vi "Measurement_input_panel.vi"(0 "OK":T4, 2 "setup":T5, 5 "Setup filename":string) -> (11 "Setup filename out":string, 12 "Analysis Info cluster":T7[](array[typedef])=[{"Colour"=0, "Inst type"=enum."Pitot-static tube", "Inst name"="Manometer voltage", "Symbol"="U", "Code name"="", "Extra Info"="U", "Inst Array"=enum."PWA", "U"=0.0, "u^2"=0.0, "u^3"=0.0, "u^4"=0.0, "Skew_u"=0.0, "Kurt_u"=0.0, "Sd Error in Mean"=0.0, "% u'/U"=0.0, "X"=0.0, "Y"=0.0, "Z"=0.0, "Timescale integral Estimate"=0.0, "Sd Error in Variance"=0.0, "Calib File"=path "", "Calib Constants"=[], "Output Position"=FALSE, "Stats"=enum."None", "Av Sampling Rate"=0.0, "Av No of Samples"=0.0, "Total Meas Time (s)"=0.0, "OrigChName"="", "Max value"=0.0, "Min value"=0.0, "Req Sample Rate Hz"=0.0, "Sync Delay Time (s)"=0.0, "Ch No"=0, "Device"="", "Use Latest Calib"=FALSE, "Port"="", "Metadata Ch Names"=[], "Metadata Ch Values"=[], "Label"="", "chState"=enum."Solo", "Point Drift"=0.0, "inputConfig"=""}, {"Colour"=0, "Inst type"=enum."Pitot-static tube", "Inst name"="Manometer voltage", "Symbol"="U", "Code name"="", "Extra Info"="U", "Inst Array"=enum."PWA", "U"=0.0, "u^2"=0.0, "u^3"=0.0, "u^4"=0.0, "Skew_u"=0.0, "Kurt_u"=0.0, "Sd Error in Mean"=0.0, "% u'/U"=0.0, "X"=0.0, "Y"=0.0, "Z"=0.0, "Timescale integral Estimate"=0.0, "Sd Error in Variance"=0.0, "Calib File"=path "", "Calib Constants"=[], "Output Position"=FALSE, "Stats"=enum."None", "Av Sampling Rate"=0.0, "Av No of Samples"=0.0, "Total Meas Time (s)"=0.0, "OrigChName"="", "Max value"=0.0, "Min value"=0.0, "Req Sample Rate Hz"=0.0, "Sync Delay Time (s)"=0.0, "Ch No"=0, "Device"="", "Use Latest Calib"=FALSE, "Port"="", "Metadata Ch Names"=[], "Metadata Ch Values"=[], "Label"="", "chState"=enum."Solo", "Point Drift"=0.0, "inputConfig"=""}, {"Colour"=0, "Inst type"=enum."Pitot-static tube", "Inst name"="Manometer voltage", "Symbol"="U", "Code name"="", "Extra Info"="U", "Inst Array"=enum."PWA", "U"=0.0, "u^2"=0.0, "u^3"=0.0, "u^4"=0.0, "Skew_u"=0.0, "Kurt_u"=0.0, "Sd Error in Mean"=0.0, "% u'/U"=0.0, "X"=0.0, "Y"=0.0, "Z"=0.0, "Timescale integral Estimate"=0.0, "Sd Error in Variance"=0.0, "Calib File"=path "", "Calib Constants"=[], "Output Position"=FALSE, "Stats"=enum."None", "Av Sampling Rate"=0.0, "Av No of Samples"=0.0, "Total Meas Time (s)"=0.0, "OrigChName"="", "Max value"=0.0, "Min value"=0.0, "Req Sample Rate Hz"=0.0, "Sync Delay Time (s)"=0.0, "Ch No"=0, "Device"="", "Use Latest Calib"=FALSE, "Port"="", "Metadata Ch Names"=[], "Metadata Ch Values"=[], "Label"="", "chState"=enum."Solo", "Point Drift"=0.0, "inputConfig"=""}] {"Kurt_u" format="%_3g"; "u^4" format="%_3g"; "u^3" format="%_3g"; "Sd Error in Variance" format="%_3g"; "u^2" format="%_3g"; "Sd Error in Mean" format="%_3g"; "U" format="%_3g"; "Sync Delay Time (s)" format="%.4f"; "Total Meas Time (s)" format="%_5g"; "Skew_u" format="%_3g"; "% u'/U" format="%_3g"})   [LabVIEW 2022 SP3]
uses:
  Controls/Inst_type.ctl
  Controls/portOrDev.ctl
  Controls/calType.ctl
  Controls/channelState.ctl
  Controls/DAQinputType.ctl
  Controls/Analysis_info_cluster.ctl
  Controls/Instrument_Array.ctl
  Controls/Setup.ctl
  Controls/ok_button.ctl
  Controls/Trigger_Mode.ctl
  Controls/PWA_Data.ctl
  File/Setup_Filetype.ctl
  Controls/Post_Process.ctl
  Controls/App_Global.ctl
  ADAM Client/Sub VIs/ADAM Controls/Channel_names.ctl
  ADAM Client/Sub VIs/Channel_State_Control.ctl
  <vilib>/Utility/error.llb/Trim Whitespace One-Sided.vi
  Globals/Meas_global.vi
  Globals/Trav_pos_global.vi
  Globals/LDA_global.vi
  Globals/Preference_global.vi
  Globals/Dynamic_call_global.ph.vi
panel:
  in  "DAQ Tigger Control?":bool
  in  "Port":refnum<visa-resource-name>="COM100"
  in  "Trigger mode":T1
  in  "Edit temp and Press":bool
  out "Abs Press":dbl=1013.0 caption="Absolute\nPressure" format="%.1fmBar"
  out "Temp":dbl=21.0 caption="Temperature" format="%.1fC"
  in  "Use  Analogue channel to software sync with LDA":bool
  in  "LDA_Setup":bool
  in  "Number of LDA Chs":i32 min=0 max=20
  in  "LDA data":enum16{"No LDA data", "Take LDA data"}(ring)=enum."Take LDA data"
  in  "PWA Data":T2
  out "Inst type":T3=enum."Propeller anemometer"
  in  "Select Plug Ins":bool
  out "XW Present?":bool
  out "Read Setup File?":bool
  out "Setup Paths":string[](array[string])
  in  "stop":bool
  out "Notes":string
  in  "Setup filename selector":u16(ring) items=["Current_Setup.xls", "GMU Source Q.xls", "7HP_Calibration.xls", "LDA_488_514_UV_Fast.xls", "LDA_488_514_UV_532_W Fast.xls", "LDA_488_514_UV_532_W.xls", "2HP_Boundary Layer.xls", "5H_Rake.xls"]
  in  "Cross wire":T6(ring)
  in  "No of Analogue inst":i32=1 caption="Number of Analogue Instruments"
  in  "Ch & spans choices":T13(array[cluster]) {"Fs" format="%#_pHz"; "syncDelay" format="%#_gms"; "Ch" min=0 step=1}
  # "Trigger Setup"
  # "Tunnel Conditions"
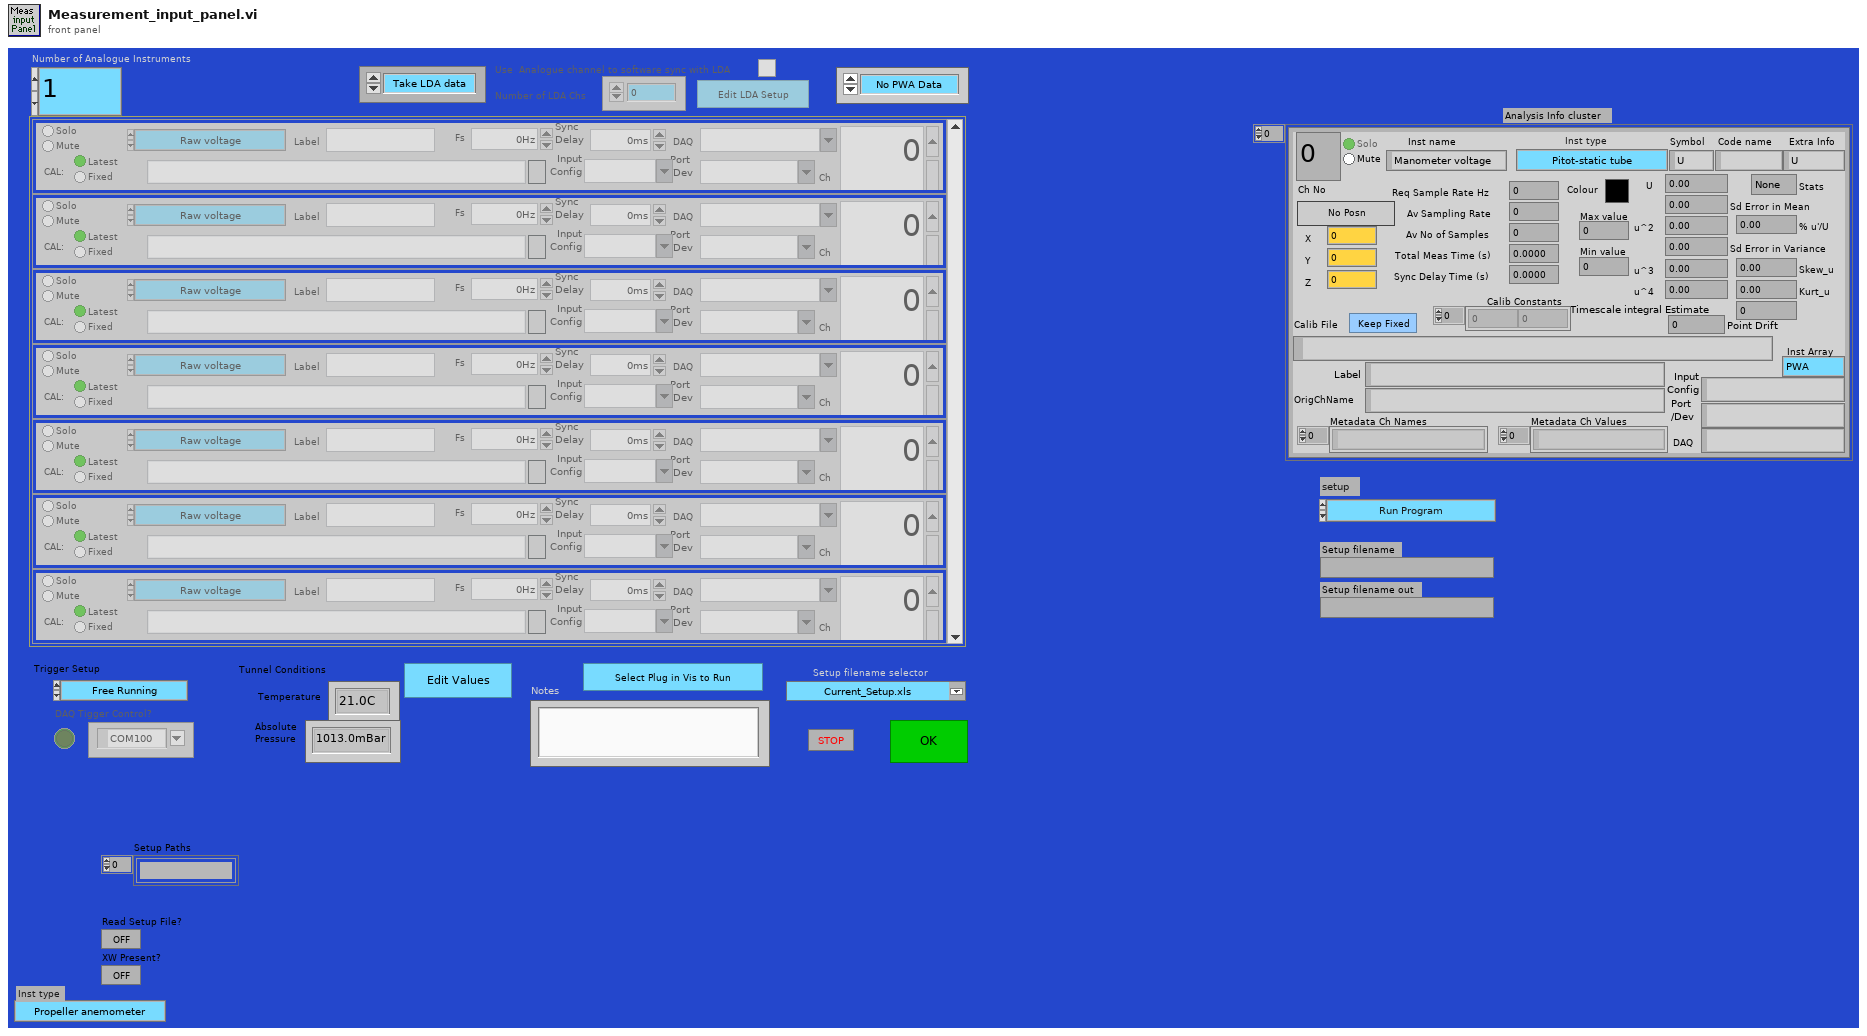
[diagram p1: front panel]
types:
  T1 = typedef "Trigger_Mode.ctl" = enum16{"Free Running", "Start on Trigger", "Trigger Every Block", "Trigger Every Sample"}
  T2 = typedef "PWA_Data.ctl" = enum16{"No PWA Data", "One Ch PWA"}
  T3 = typedef "Inst_type.ctl" = enum16{"Raw voltage", "Raw with zero offsetting", "Propeller anemometer", "Pressure Transducer", "Pitot-static tube", "Hot wire", "Cross wire 1", "Cross wire 2", "Generic Linear", "Generic Polynomial", "Generic BackPoly", "Fast FID", "Thermocouple", "Cold wire", "Pulsed Wire", "LDA Vel", "LDA Tran time", "LDA Arr time", "Microphone"}
  T4 = typedef "ok_button.ctl" = bool
  T5 = typedef "Setup.ctl" = enum16{"Run Program", "Show Setup", "Save Current Setup", "Setup Front Panel"}
  T6 = enum16{"2nd component as calculated", "2nd component multipled by -1"}
  T7 = typedef "Analysis_info_cluster.ctl" = cluster{"Colour":u32, "Inst type":T3, "Inst name":string, "Symbol":string, "Code name":string, "Extra Info":string, "Inst Array":T8, "U":dbl, "u^2":dbl, "u^3":dbl, "u^4":dbl, "Skew_u":dbl, "Kurt_u":dbl, "Sd Error in Mean":dbl, "% u'/U":dbl, "X":dbl, "Y":dbl, "Z":dbl, "Timescale integral Estimate":dbl, "Sd Error in Variance":dbl, "Calib File":path, "Calib Constants":dbl[], "Output Position":bool, "Stats":enum16{"None", "Basic", "Full"}, "Av Sampling Rate":dbl, "Av No of Samples":dbl, "Total Meas Time (s)":dbl, "OrigChName":string, "Max value":dbl, "Min value":dbl, "Req Sample Rate Hz":dbl, "Sync Delay Time (s)":dbl, "Ch No":i16, "Device":string, "Use Latest Calib":bool, "Port":string, "Metadata Ch Names":string[], "Metadata Ch Values":string[], "Label":string, "chState":T9, "Point Drift":dbl, "inputConfig":string}
  T8 = typedef "Instrument_Array.ctl" = enum16{"PWA", "LDA", "Analogue"}
  T9 = typedef "channelState.ctl" = enum32{"No Selection", "Solo", "Mute"}
  T10 = typedef "portOrDev.ctl" = string
  T11 = typedef "calType.ctl" = enum32{"Latest", "Fixed"}
  T12 = typedef "DAQinputType.ctl" = string
  T13 = cluster{"Type":T3, "Label":string, "DAQ":string, "Port":T10, "Ch":i32, "Cal":path, "calType":T11, "Fs":dbl, "syncDelay":dbl, "chState":T9, "inputConfig":T12}[]
  T14 = typedef "Post_Process.ctl" = enum16{"Take New Data", "Post Process Raw Data File"}
  T15 = typedef "Setup_Filetype.ctl" = enum16{"Measurement Setups", "Calibration Setups", "General", "Results File Plotter Setups", "Speed Calib Tweaks"}
  T16 = enum8{"Enabled", "Disabled", "Disabled and Grayed Out"}
  T17 = typedef "App_Global.ctl" = enum16{"Read Global", "Write to Global", "Initialise Array"}
  T18 = typedef "Channel_names.ctl" = enum16{"Active Only", "Active + Off", "All Channels", "Changeable Only", "Always Off", "Always On", "Always Off or On"}
  T19 = typedef "Channel_State_Control.ctl" = enum16{"Channel Name", "Channel Name Starts with", "Main Address"}
  T20 = enum16{"Zero or one", "One", "Zero or more", "One or more"}
  T21 = typedef "Meas input Cluster.ctl" = cluster{"Type":T3, "Label":string, "DAQ":string, "Port":T10, "Ch":i32, "Cal":path, "calType":T11, "Fs":dbl, "syncDelay":dbl, "chState":T9, "inputConfig":T12}
  T22 = typedef "LDA_Channel.ctl" = cluster{"Wavelength (nm)":dbl, "Vel Comp":string, "Max Velocity":dbl, "Min Velocity":dbl, "Max Record length":u16, "Signal gain (dB)":i16, "High voltage":i16, "Optics Conversion Factor":dbl, "Min Record length":u16, "Multiply Velocity by -1":bool, "Signal to Noise Ratio":string, "Validation Ratio":string, "Probe":string, "Laser":string, "BSA":string, "Lense":string, "Beam Separation (mm)":dbl, "Focal Length (mm)":dbl, "COLOUR":u32, "BSA IP":string, "Velocity Range (m/s)":dbl, "Centre Velocity (m/s)":dbl, "Unshifted mW":dbl, "Shifted mW":dbl, "Bandwidth Hz":dbl, "Req Sampling Rate Hz":dbl, "Ch":i32, "CenterFreq Hz":dbl, "Laser IP":string, "Sync Delay (s)":dbl}
  T23 = cluster{"Type":T3, "Label":string, "DAQ":string, "Port":T10, "Ch":i32, "Cal":path, "calType":T11, "Fs":dbl, "syncDelay":dbl, "chState":T9, "inputConfig":T12}
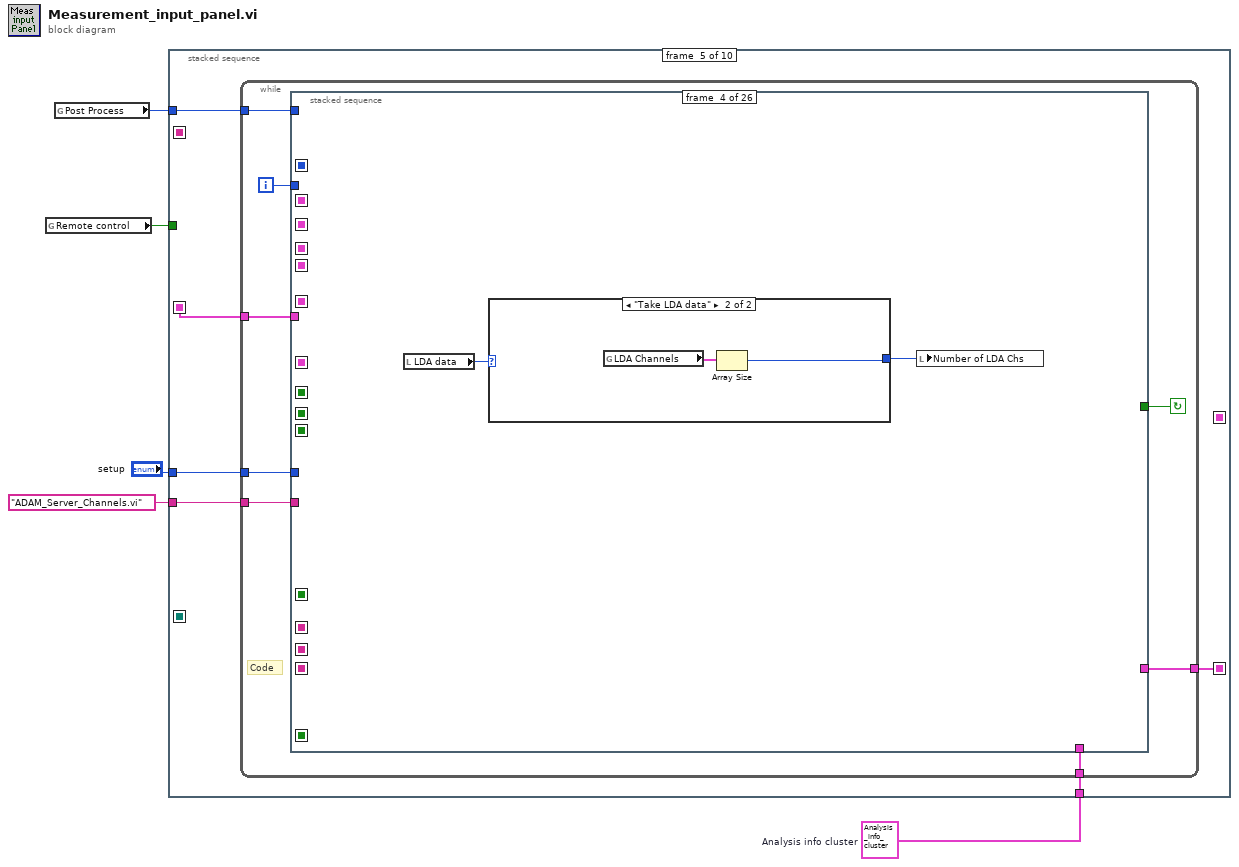
[diagram p0: block diagram]
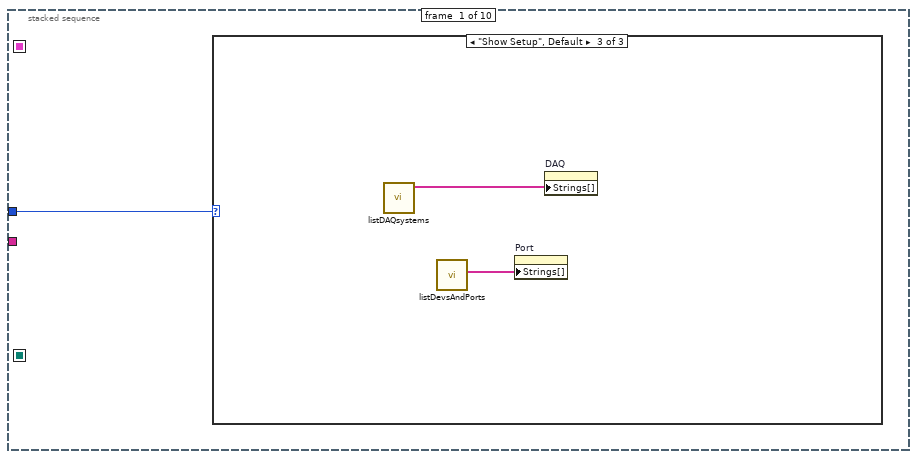
[diagram p2: hidden frame]
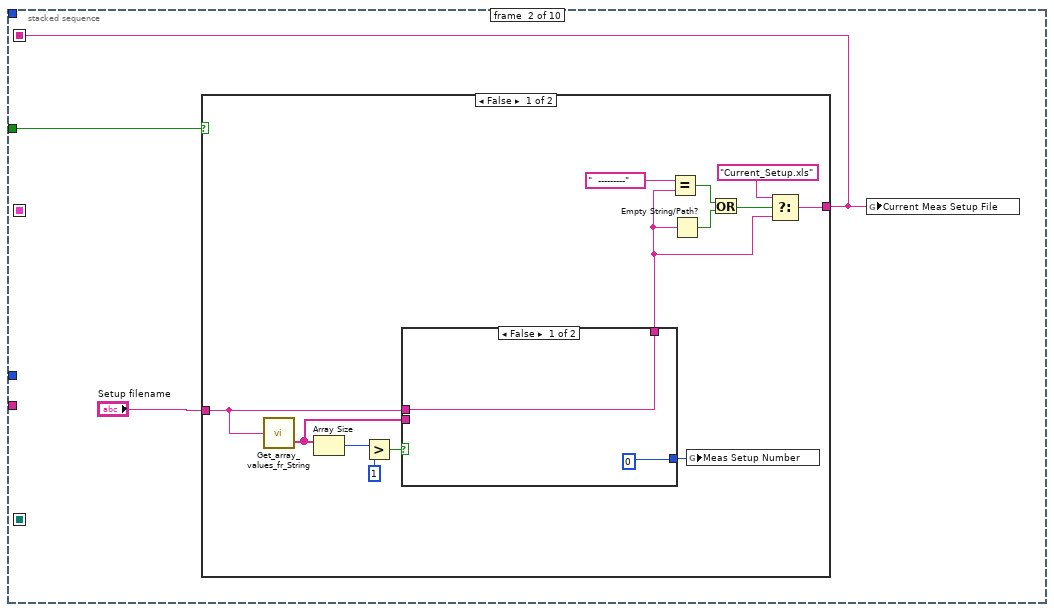
[diagram p5: hidden frame]
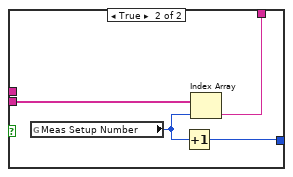
[diagram p6: hidden frame]
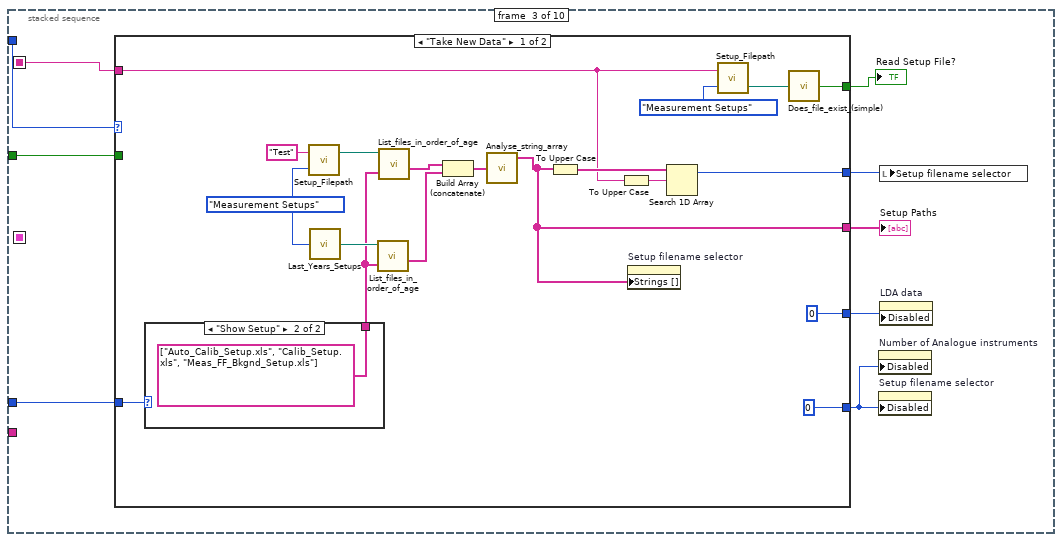
[diagram p8: hidden frame]
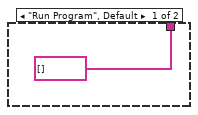
[diagram p9: hidden frame]
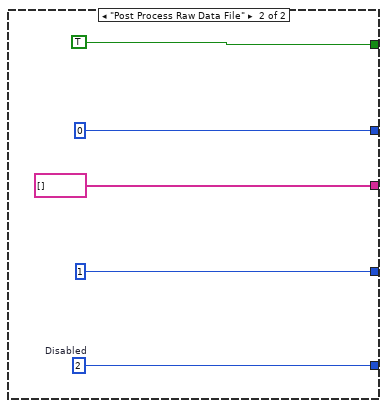
[diagram p10: hidden frame]
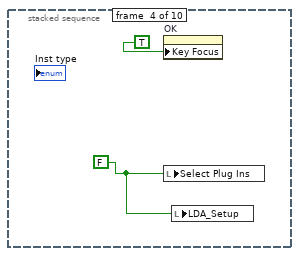
[diagram p11: hidden frame]
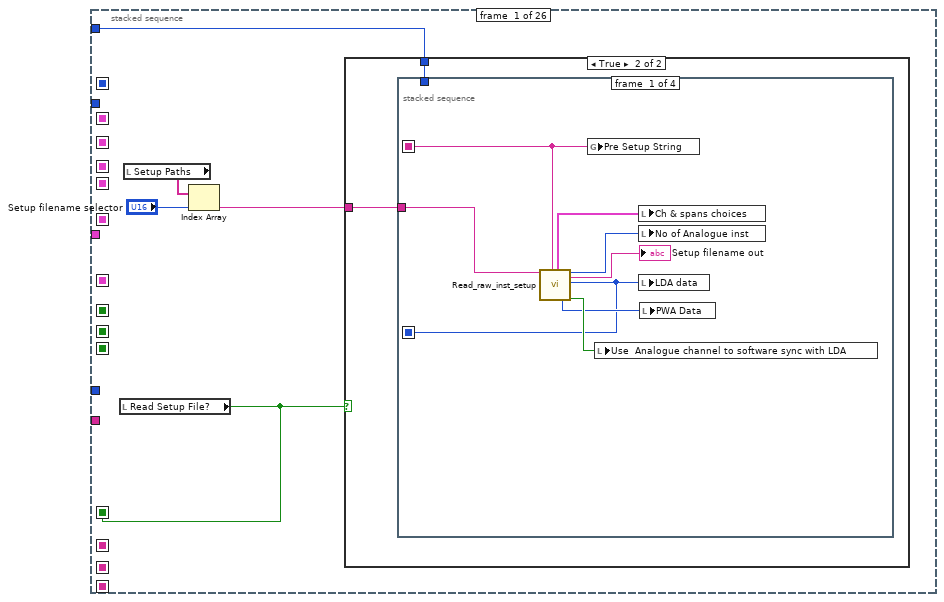
[diagram p12: hidden frame]
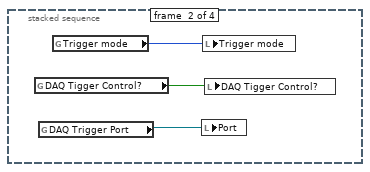
[diagram p14: hidden frame]
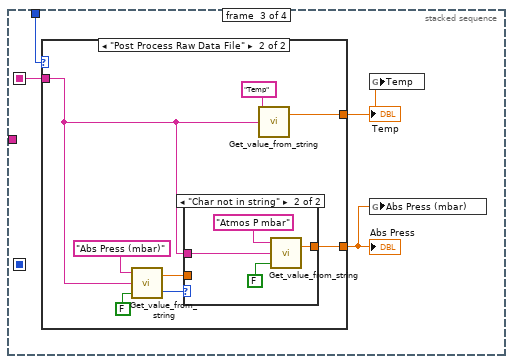
[diagram p15: hidden frame]
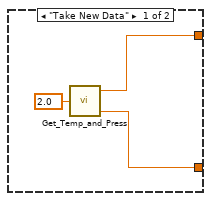
[diagram p16: hidden frame]
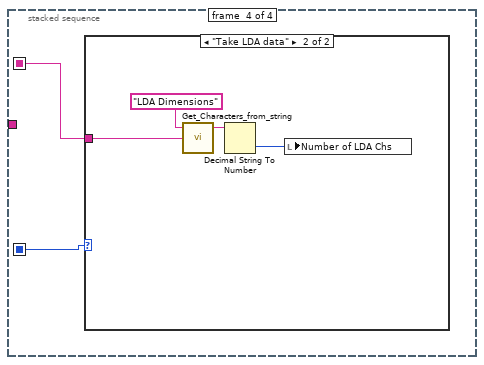
[diagram p18: hidden frame]
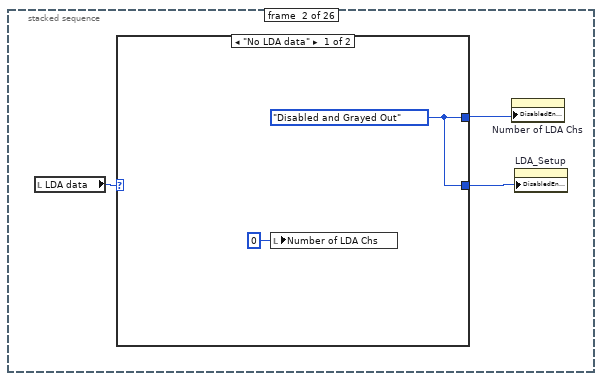
[diagram p20: hidden frame]
diagram:
  w1 = T7 {"Colour"=0, "Inst type"=enum."Pitot-static tube", "Inst name"="Manometer voltage", "Symbol"="U", "Code name"="", "Extra Info"="U", "Inst Array"=enum."PWA", "U"=0.0, "u^2"=0.0, "u^3"=0.0, "u^4"=0.0, "Skew_u"=0.0, "Kurt_u"=0.0, "Sd Error in Mean"=0.0, "% u'/U"=0.0, "X"=0.0, "Y"=0.0, "Z"=0.0, "Timescale integral Estimate"=0.0, "Sd Error in Variance"=0.0, "Calib File"=path "", "Calib Constants"=[], "Output Position"=FALSE, "Stats"=enum."None", "Av Sampling Rate"=0.0, "Av No of Samples"=0.0, "Total Meas Time (s)"=0.0, "OrigChName"="", "Max value"=0.0, "Min value"=0.0, "Req Sample Rate Hz"=0.0, "Sync Delay Time (s)"=0.0, "Ch No"=0, "Device"="", "Use Latest Calib"=FALSE, "Port"="", "Metadata Ch Names"=[], "Metadata Ch Values"=[], "Label"="", "chState"=enum."Solo", "Point Drift"=0.0, "inputConfig"=""}  # Analysis info cluster
  n1 = global read "Meas_global.vi" "Remote control"() -> (w3:bool)
  n2 = global read "Meas_global.vi" "Post Process"() -> (w5:T14)
  n3 = stacked-sequence {
    seq-local: [_ _ _ _ w74 _ _ _ _ _] -> [_ _ _ _ _ _ _ w765 _ _]
    seq-local: [_ w10 _ _ _ _ _ _ _ _] -> [_ _ w32 _ _ _ w630 _ _ _]
    seq-local: [_ _ _ _ w71 _ _ _ _ _] -> [_ _ _ _ _ _ _ _ _ w860]
    seq-local: [_ _ _ _ _ _ _ w764 _ _] -> [_ _ _ _ _ _ _ _ _ w861]
    seq-local: [_ _ _ _ _ _ _ _ w823 _] -> [_ _ _ _ _ _ _ _ _ w864]
    tunnel: w5 -> [_ _ w40 _ w73 _ _ w766 _ _]
    tunnel: "setup" -> [w6 _ w34 _ w72 _ w631 _ _ _]
    tunnel: w3 -> [_ w11 w33 _ _ _ _ _ _ _]
    tunnel: "ADAM_Server_Channels.vi" -> [_ _ _ _ w70 _ _ _ _ _]
    tunnel: w1 -> [_ _ _ _ w69 _ _ _ w826 _]
    frame #0 {
      n4 = case shown="\"Show Setup\", Default" w6 {
        frame "Run Program" {
        }
        frame "Setup Front Panel" {
        }
        frame "Show Setup", Default {
          n5 = call "listDAQsystems.vi"() -> ("DAQsystems"=w7:string[])  [unwired: 11 in]
          n6 = call "listDevsAndPorts.vi"() -> ("All Available Ports"=w8:string[])  [unwired: 11 in]
          n7 = property on="Port" class="CmbBox (strict)"("Strings[]"=w8) -> ()  [unwired: 2 in, 2 out]
          n8 = property on="DAQ" class="CmbBox"("Strings[]"=w7) -> ()  [unwired: 2 in, 2 out]
        }
      }
    }
    frame #1 {
      n9 = case shown="False" w11 {
        tunnel: [w23 w31] -> w10
        tunnel: "Setup filename" -> [w12 w31]
        frame False {
          n10 = call "Get_array_values_fr_String.vi"("String Value"=w12) -> ("String array"=w14:string[])  [unwired: 1 out]
          n11 = Array Size(array=w14) -> (size(s)=w18:i32)
          n12 = Greater?(x=w18, y=1) -> (0:w16:bool)
          n13 = case shown="False" w16 {
            tunnel: [w26 w29] -> w15
            tunnel: w12 -> [w26 _]
            tunnel: w14 -> [_ w30]
            tunnel: [0 w27] -> w13
            frame False {
            }
            frame True {
              n14 = global read "Trav_pos_global.vi" "Meas Setup Number"() -> (w28:i32)
              n15 = Increment(x=w28) -> (x+1=w27:i32)
              n16 = Index Array(array=w30, index=w28) -> (element=w29:string)
            }
          }
          n17 = Equal?(x="  ---------" ("f"), y=w15) -> (x = y?=w22:bool)
          n18 = Empty String/Path?(string/path=w15) -> (empty?=w21:bool)
          n19 = global write "Trav_pos_global.vi" "Meas Setup Number"(w13) -> ()
          n20 = Or(x=w22, y=w21) -> (x .or. y?=w19:bool)
          n21 = Select(t="Current_Setup.xls", s=w19, f=w15) -> (s? t:f=w23:string)
        }
        frame True {
        }
      }
      n22 = global write "Trav_pos_global.vi" "Current Meas Setup File"(w10) -> ()
    }
    frame #2 {
      n23 = case shown="\"Take New Data\"" w40 {
        tunnel: [w41 string[] []] -> w36
        tunnel: [w55 TRUE ("exists")] -> w35
        tunnel: [u8 0 ("Disabled") w63] -> w37
        tunnel: [u8 0 ("Disabled") u8 1 ("Disabled")] -> w39
        tunnel: w32 -> [w51 _]
        tunnel: [w58 0 ("index of element")] -> w38
        tunnel: w34 -> [w53 _]
        tunnel: w33 -> [_ _]
        frame "Take New Data" {
          w45 = Setup_Filetype."Measurement Setups" ("Setup File Type")
          n24 = case shown="\"Show Setup\"" w53 {
            tunnel: [string[] [] ("file names") string[] ["Auto_Calib_Setup.xls", "Calib_Setup.xls", "Meas_FF_Bkgnd_Setup.xls"] ("file names")] -> w43
            frame "Run Program", Default {
            }
            frame "Show Setup" {
            }
          }
          n25 = call "Setup_Filepath.vi"("Setup File Type"=w45, "Filename in"="Test") -> ("Directory"=w46:path)  [unwired: 1 out]
          n26 = call "Last_Years_Setups.vi"("Setup File Type"=w45) -> ("Directory"=w44:path)
          n27 = call "List_files_in_order_of_age.vi"("Files to Hide"=w43, "Folder"=w44) -> ("file names"=w48:string[])  [unwired: 9 in]
          n28 = call "List_files_in_order_of_age.vi"("Files to Hide"=w43, "Folder"=w46) -> ("file names"=w47:string[])  [unwired: 9 in]
          n29 = Build Array (concatenate)(w47, w48) -> (w42:string[])
          n30 = call "Analyse_string_array.vi"("String array"=w42) -> ("Unique strings"=w41:string[])  [unwired: 1 in, 1 out]
          n31 = To Upper Case(1:w41) -> (0:w57:string[])
          n32 = To Upper Case(1:w51) -> (0:w56:string)
          n33 = property on="Setup filename selector" class="Ring (strict)"("Strings []"=w41) -> ()  [unwired: 2 in, 2 out]
          n34 = Search 1D Array(1D array=w57, element=w56) -> (index of element=w58:i32)  [unwired: 1 out]
          n35 = call "Setup_Filepath.vi"("Setup File Type"=Setup_Filetype."Measurement Setups", "Filename in"=w51) -> ("Filename Out"=w50:path)  [unwired: 1 out]
          n36 = call "Does_file_exist_(simple).vi"("Pathname"=w50) -> ("exists?"=w55:bool)
        }
        frame "Post Process Raw Data File" {
          w63 = u8 2  # Disabled
        }
      }
      "Setup Paths" <- w36
      "Read Setup File?" <- w35
      n37 = property on="Number of Analogue instruments" class="DigNum (strict)"("Disabled"=w37) -> ()  [unwired: 2 in, 2 out]
      n38 = property on="Setup filename selector" class="Ring (strict)"("Disabled"=w37) -> ()  [unwired: 2 in, 2 out]
      n39 = local write "Setup filename selector"(w38) -> ()
      n40 = property on="LDA data" class="Enum (strict)"("Disabled"=w39) -> ()  [unwired: 2 in, 2 out]
    }
    frame #3 {
      w67 = FALSE ("Select Local ADAM Channels")
      n41 = property on="OK" class="Bool"("Key Focus"=TRUE) -> ()  [unwired: 2 in, 2 out]
      n42 = local write "Select Plug Ins"(w67) -> ()
      n43 = local write "LDA_Setup"(w67) -> ()
    }
    frame #4 {
      n44 = while {
        tunnel: w72 -> [w79]
        tunnel: w73 -> [w80]
        tunnel: [w82] -> w74
        tunnel: [w78] -> w71
        tunnel: w70 -> [w77]
        tunnel: w69 -> [w75]
        i -> [w76]
        stop <- w81 continue-if-true
        # "Code"
        n45 = stacked-sequence {
          seq-local: [_ _ _ _ _ _ _ _ _ _ _ w229 _ _ _ _ _ _ _ _ _ _ _ _ _ _] -> [_ _ _ _ _ _ _ _ _ _ _ _ _ _ w293 w346 _ _ _ _ _ _ _ _ _ _]
          seq-local: [_ _ _ _ "Ch & spans choices" _ _ _ _ _ _ _ _ _ _ _ _ _ _ _ _ _ _ _ _ _] -> [_ _ _ _ _ w168 _ _ w193 _ w225 w230 _ _ _ _ _ _ _ _ _ w566 _ _ _ _]
          seq-local: [_ _ _ _ _ _ _ _ w198 _ _ _ _ _ _ _ _ _ _ _ _ _ _ _ _ _] -> [_ _ _ _ _ _ _ _ _ _ _ w231 _ _ _ _ _ _ _ _ _ _ _ _ _ _]
          seq-local: [_ _ _ _ _ _ _ _ _ _ _ _ _ "OK" _ _ _ _ _ _ _ _ _ _ _ _] -> [_ _ _ _ _ _ _ _ _ _ _ _ _ _ w292 _ _ _ _ _ _ _ _ _ _ w595]
          seq-local: [_ _ _ _ _ _ _ _ _ _ _ _ _ _ _ _ w383 _ _ _ _ _ _ _ _ _] -> [_ _ _ _ _ _ _ _ _ _ _ _ _ _ _ _ _ _ w411 _ _ _ _ _ _ _]
          seq-local: [_ _ _ _ _ _ _ _ _ _ _ _ _ _ w297 _ _ _ _ _ _ _ _ _ _ _] -> [_ _ _ _ _ _ _ _ _ _ _ _ _ _ _ _ w385 _ _ _ _ _ _ _ _ _]
          seq-local: [_ _ _ _ _ _ _ _ _ _ _ _ _ _ _ w345 _ _ _ _ _ _ _ _ _ _] -> [_ _ _ _ _ _ _ _ _ _ _ _ _ _ _ _ w384 _ _ _ _ _ _ _ _ _]
          seq-local: [_ _ _ _ _ _ _ _ _ _ _ _ w287 _ _ _ _ _ _ _ _ _ _ _ _ _] -> [_ _ _ _ _ _ _ _ _ _ _ _ _ _ w294 _ _ _ _ _ _ _ _ _ _ w594]
          seq-local: [_ _ _ _ _ _ _ _ _ _ _ _ _ _ _ _ _ _ _ w458 _ _ _ _ _ _] -> [_ _ _ _ _ _ _ _ _ _ _ _ _ _ _ _ _ _ _ _ w536 _ _ _ _ _]
          seq-local: [_ _ _ _ _ _ _ _ _ _ _ _ _ _ _ _ _ _ _ w453 _ _ _ _ _ _] -> [_ _ _ _ _ _ _ _ _ _ _ _ _ _ _ _ _ _ _ _ w535 _ _ _ _ _]
          seq-local: [_ _ _ _ _ _ _ _ _ _ _ _ _ _ _ _ _ _ _ w457 _ _ _ _ _ _] -> [_ _ _ _ _ _ _ _ _ _ _ _ _ _ _ _ _ _ _ _ w534 _ _ _ _ _]
          seq-local: [w83 _ _ _ _ _ _ _ _ _ _ _ _ _ _ _ _ _ _ _ _ _ _ _ _ _] -> [_ _ _ _ _ _ _ _ _ _ _ _ _ _ _ _ _ _ _ _ w532 _ _ _ _ _]
          seq-local: [_ _ _ _ _ _ _ _ _ _ _ _ _ _ _ _ _ _ w412 _ _ _ _ _ _ _] -> [_ _ _ _ _ _ _ _ _ _ _ _ _ _ _ _ _ _ _ w455 _ w567 _ w570 _ w587]
          seq-local: [_ _ _ _ _ _ _ _ _ _ _ _ _ _ _ _ _ w403 _ _ _ _ _ _ _ _] -> [_ _ _ _ _ _ _ _ _ _ _ _ _ _ _ _ _ _ w413 _ _ _ _ _ _ _]
          seq-local: [_ _ _ _ _ _ _ _ _ _ _ _ _ _ _ _ _ _ _ w454 _ _ _ _ _ _] -> [_ _ _ _ _ _ _ _ _ _ _ _ _ _ _ _ _ _ _ _ w530 _ _ _ _ _]
          tunnel: [_ _ _ _ _ _ _ _ _ _ _ _ _ _ _ _ w383 _ _ _ _ _ _ _ _ _] -> w82
          tunnel: [_ _ _ _ _ _ _ _ _ _ _ _ _ _ w295 _ _ _ _ _ _ _ _ _ _ _] -> w81
          tunnel: w80 -> [w85 _ _ _ _ _ w174 _ _ _ _ _ w288 _ _ w344 _ w409 _ _ _ _ _ _ _ _]
          tunnel: w79 -> [_ _ _ _ _ w167 _ w181 _ _ _ _ _ _ _ _ w386 _ _ _ _ _ _ _ _ _]
          tunnel: [_ _ _ _ _ _ _ _ _ _ _ _ _ _ _ _ _ _ _ _ w533 _ _ _ _ _] -> w78
          tunnel: w77 -> [_ _ _ _ _ _ _ _ _ _ _ _ _ _ w291 _ _ w406 w414 _ _ _ _ _ _ _]
          tunnel: w76 -> [_ _ _ _ _ _ _ _ _ _ _ _ _ _ _ _ _ _ _ _ _ _ _ _ _ _]
          tunnel: w75 -> [_ _ _ _ _ _ _ _ _ _ _ _ _ _ _ _ _ _ _ _ w531 _ _ _ _ _]
          frame #0 {
            n46 = local read "Read Setup File?"() -> (w83:bool)
            n47 = local read "Setup Paths"() -> (w87:string[])
            n48 = Index Array(array=w87, index="Setup filename selector") -> (element=w84:string)
            n49 = case shown="True" w83 {
              tunnel: w84 -> [_ w89]
              tunnel: w85 -> [_ w88]
              frame False {
              }
              frame True {
                n50 = stacked-sequence {
                  seq-local: [w94 _ _ _] -> [_ _ w103 w121]
                  seq-local: [w92 _ _ _] -> [_ _ _ w122]
                  tunnel: w89 -> [w95 _ _ _]
                  tunnel: w88 -> [_ _ w104 _]
                  frame #0 {
                    n51 = call "Read_raw_inst_setup.vi"("Setup file"=w95) -> ("Setup string"=w94:string, "Ch & spans choices"=w91:T21[], "PWA Data"=w93:T2, "Number of Analogue instruments"=w97:i32, "Setup filename out"=→"Setup filename out":string, "LDA data"=w92:enum16{"No LDA data", "Take LDA data"}, "Use Analogue channel to software sync with LDA"=w96:bool)  [unwired: 12 out]
                    n52 = global write "Meas_global.vi" "Pre Setup String"(w94) -> ()
                    n53 = local write "Use  Analogue channel to software sync with LDA"(w96) -> ()
                    n54 = local write "Ch & spans choices"(w91) -> ()
                    n55 = local write "No of Analogue inst"(w97) -> ()
                    n56 = local write "LDA data"(w92) -> ()
                    n57 = local write "PWA Data"(w93) -> ()
                  }
                  frame #1 {
                    n58 = global read "Meas_global.vi" "DAQ Tigger Control?"() -> (w98:bool)
                    n59 = global read "Meas_global.vi" "DAQ Trigger Port"() -> (w99:refnum<visa-resource-name>)
                    n60 = global read "Meas_global.vi" "Trigger mode"() -> (w100:T1)
                    n61 = local write "Port"(w99) -> ()
                    n62 = local write "Trigger mode"(w100) -> ()
                    n63 = local write "DAQ Tigger Control?"(w98) -> ()
                  }
                  frame #2 {
                    n64 = case shown="\"Post Process Raw Data File\"" w104 {
                      tunnel: w103 -> [_ w110]
                      tunnel: [w105 w109] -> w101
                      tunnel: [w106 w108] -> w102
                      frame "Take New Data" {
                        n65 = call "Get_Temp_and_Press.vi"("Averaging time (mins)"=2.0) -> ("Abs Press (mbar)"=w105:dbl, "Temperature"=w106:dbl)  [unwired: 3 out]
                      }
                      frame "Post Process Raw Data File" {
                        n66 = call "Get_value_from_string.vi"("Show Dialog?"=FALSE, "Input string"=w110, "Variable name"="Abs Press (mbar)") -> ("Status"=w114:enum16{"Char in string", "Char not in string"}, "Value"=w113:dbl)
                        n67 = case shown="\"Char not in string\"" w114 {
                          tunnel: [w116 w119] -> w109
                          tunnel: w113 -> [w116 _]
                          tunnel: w110 -> [_ w118]
                          frame "Char in string" {
                          }
                          frame "Char not in string" {
                            n68 = call "Get_value_from_string.vi"("Show Dialog?"=FALSE, "Input string"=w118, "Variable name"="Atmos P mbar") -> ("Value"=w119:dbl)  [unwired: 1 out]
                          }
                        }
                        n69 = call "Get_value_from_string.vi"("Input string"=w110, "Variable name"="Temp") -> ("Value"=w108:dbl)  [unwired: 1 in, 1 out]
                      }
                    }
                    "Abs Press" <- w101
                    "Temp" <- w102
                    n70 = global write "Meas_global.vi" "Temp"(w102) -> ()
                    n71 = global write "Meas_global.vi" "Abs Press (mbar)"(w101) -> ()
                  }
                  frame #3 {
                    n72 = case shown="\"Take LDA data\"" w122 {
                      tunnel: w121 -> [_ w124]
                      frame "No LDA data" {
                      }
                      frame "Take LDA data" {
                        n73 = call "Get_Characters_from_string.vi"("Input string"=w124, "Variable name"="LDA Dimensions") -> ("Value"=w126:string)  [unwired: 1 in, 1 out]
                        n74 = Decimal String To Number(string=w126) -> (number=w123:i32)  [unwired: 2 in, 1 out]
                        n75 = local write "Number of LDA Chs"(w123) -> ()
                      }
                    }
                  }
                }
              }
            }
          }
          frame #1 {
            n76 = local read "LDA data"() -> (w129:enum16{"No LDA data", "Take LDA data"})
            n77 = case shown="\"No LDA data\"" w129 {
              tunnel: [w130 w132] -> w128
              tunnel: [w130 w132] -> w127
              frame "No LDA data" {
                w130 = T16."Disabled and Grayed Out" ("Disabled")
                n78 = local write "Number of LDA Chs"(i16 0 ("Number of LDA Chs")) -> ()
              }
              frame "Take LDA data" {
                w132 = T16."Enabled" ("Disabled")
              }
            }
            n79 = property on="Number of LDA Chs" class="DigNum (strict)"("DisabledEnum"=w128) -> ()  [unwired: 2 in, 2 out]
            n80 = property on="LDA_Setup" class="Bool (strict)"("DisabledEnum"=w127) -> ()  [unwired: 2 in, 2 out]
          }
          frame #2 {
            n81 = case shown="True" "LDA_Setup" {
              frame False {
              }
              frame True {
                n82 = global read "Meas_global.vi" "Pre Setup String"() -> (w137:string)
                n83 = call "Get_value_from_string.vi"("Input string"=w137, "Variable name"="BSA 1 Calibration factor") -> ("Status"=w136:enum16{"Char in string", "Char not in string"})  [unwired: 1 in, 1 out]
                n84 = local write "LDA_Setup"(FALSE ("LDA_Setup")) -> ()
                n85 = Equal?(x=w136, y=enum16{"Char in string", "Char not in string"}."Char in string" ("Status")) -> (x = y?=w134:bool)
                n86 = call "Edit LDA Setup.vi"("LDA info in Setup File?"=w134) -> ()  [unwired: 11 in]
              }
            }
          }
          frame #3 {
            n87 = local read "LDA data"() -> (w141:enum16{"No LDA data", "Take LDA data"})
            n88 = case shown="\"Take LDA data\"" w141 {
              tunnel: [0 ("Number of LDA Chs") w143] -> w140
              frame "No LDA data" {
              }
              frame "Take LDA data" {
                n89 = global read "LDA_global.vi" "LDA Channels"() -> (w144:T22[])
                n90 = Array Size(array=w144) -> (size(s)=w143:i32)
              }
            }
            n91 = local write "Number of LDA Chs"(w140) -> ()
          }
          frame #4 {
            n92 = local read "Read Setup File?"() -> (w150:bool)
            n93 = local read "Trigger mode"() -> (w148:T1)
            n94 = case shown="True" w150 {
              frame False {
              }
              frame True {
                n95 = global read "Meas_global.vi" "Pre Setup String"() -> (w159:string)
                n96 = call "Get_Characters_from_string.vi"("Input string"=w159, "Variable name"="Invert Second Component") -> ("Status"=w158:enum16{"Char in string", "Char not in string"}, "Value"=w157:string)  [unwired: 1 in]
                n97 = case shown="\"Char in string\"" w158 {
                  tunnel: w157 -> [w166 _]
                  frame "Char in string" {
                    n98 = Equal?(x="TRUE", y=w166) -> (x = y?=w162:bool)
                    n99 = Select(t=T6."2nd component multipled by -1" ("Cross wire/LDA"), s=w162, f=T6."2nd component as calculated" ("Cross wire/LDA")) -> (s? t:f=w164:T6)
                    n100 = local write "Cross wire"(w164) -> ()
                  }
                  frame "Char not in string" {
                  }
                }
              }
            }
            n101 = case shown="Default" w148 {
              tunnel: [w151 w152] -> w147
              tunnel: [w151 w153] -> w146
              tunnel: "DAQ Tigger Control?" -> [_ w154]
              frame "Free Running" {
                w151 = T16."Disabled and Grayed Out" ("Disabled")
              }
              frame Default {
                w152 = T16."Enabled" ("Disabled")
                n102 = case shown="False" w154 {
                  tunnel: [T16."Disabled and Grayed Out" ("Disabled") w156] -> w153
                  tunnel: w152 -> [_ w156]
                  frame False {
                  }
                  frame True {
                  }
                }
              }
            }
            n103 = property on="Port" class="VISAName"("DisabledEnum"=w146) -> ()  [unwired: 2 in, 2 out]
            n104 = property on="DAQ Tigger Control?" class="Bool (strict)"("DisabledEnum"=w147) -> ()  [unwired: 2 in, 2 out]
          }
          frame #5 {
            n105 = case shown="\"Show Setup\"" w167 {
              tunnel: w168 -> [_ w171]
              frame "Run Program", Default {
              }
              frame "Show Setup" {
                n106 = for {
                  tunnel: w171 -> [w173] mode=indexing
                  tunnel: [w172] -> w170 mode=indexing
                  n107 = Unbundle By Name(w173) -> ("DAQ"=w172:string)
                }
                n108 = call "Analyse_string_array.vi"("String array"=w170) -> ("Unique strings"=w169:string[])  [unwired: 1 in, 1 out]
                n109 = global write "Meas_global.vi" "Acquisition_Plug_Ins to Run"(w169) -> ()
              }
            }
          }
          frame #6 {
            n110 = case shown="True" "Edit temp and Press" {
              tunnel: w174 -> [_ w176]
              frame False {
              }
              frame True {
                n111 = case shown="\"Take New Data\"" w176 {
                  frame "Take New Data" {
                    n112 = stacked-sequence {
                      frame #0 {
                        w177 = TRUE  # Wait until done
                        n113 = call "Run_Enter_Temp.vi"("Wait until done"=w177) -> ()  [unwired: 1 out]
                      }
                      frame #1 {
                        n114 = call "Get_Temp_and_Press.vi"("Averaging time (mins)"=2.0) -> ("Abs Press (mbar)"=w178:dbl, "Temperature"=w179:dbl)  [unwired: 3 out]
                        n115 = local write "Abs Press"(w178) -> ()
                        n116 = local write "Temp"(w179) -> ()
                      }
                    }
                  }
                  frame "Post Process Raw Data File" {
                  }
                }
              }
            }
          }
          frame #7 {
            n117 = case shown="True" "Select Plug Ins" {
              tunnel: w181 -> [_ w183]
              frame False {
              }
              frame True {
                n118 = stacked-sequence {
                  tunnel: w183 -> [w184 _]
                  frame #0 {
                    w188 = TRUE  # Show Panel?
                    n119 = global read "Meas_global.vi" "Pre Setup String"() -> (w187:string)
                    n120 = local write "Select Plug Ins"(FALSE ("Select Local ADAM Channels")) -> ()
                    n121 = call "Choose_Plug_In_to_Run.vi"("setup"=w184, "Show Panel?"=w188, "Setup String In"=w187) -> ("Setup String Out"=w186:string)  [unwired: 1 out]
                    n122 = global write "Meas_global.vi" "Pre Setup String"(w186) -> ()
                  }
                  frame #1 {
                    n123 = Current VI's Path() -> (path=w190:path)
                    n124 = call "Open_Close_Front_Panel.ph.vi"("openWindow (T)"=TRUE ("Front Panel Window:Open"), "VI path"=w190) -> ()  [unwired: 1 in, 1 out]
                  }
                }
              }
            }
          }
          frame #8 {
            n125 = Initialize Array(0) -> (w200:i32[])  [unwired: 1 out]
            n126 = for {
              shift-right: [w205] -> w196
              shift-left: w200 -> [w206]
              tunnel: [w204] -> w194 mode=indexing
              tunnel: w193 -> [w203] mode=indexing
              n127 = Unbundle By Name(w203) -> ("Type"=w202:T3)
              n128 = case shown="\"LDA Vel\"" w202 {
                tunnel: w206 -> [w210 w214 w216 w220]
                tunnel: [w209 w213 w216 w219] -> w205
                tunnel: [FALSE TRUE FALSE FALSE] -> w204
                frame "Propeller anemometer", Default {
                  n129 = Build Array (concatenate)(w210, 1) -> (w209:i32[])
                }
                frame "Cross wire 1" {
                  n130 = Build Array (concatenate)(w214, 2) -> (w213:i32[])
                }
                frame "Cross wire 2" {
                }
                frame "LDA Vel" {
                  n131 = Build Array (concatenate)(w220, 1) -> (w219:i32[])
                }
              }
            }
            n132 = Or Array Elements(Boolean array=w194) -> (logical OR=→"XW Present?":bool)
            n133 = Build Array (concatenate)(w196, 1) -> (w195:i32[])
            n134 = Array Subset(array=w195, length="No of Analogue inst") -> (w199:i32[])  [unwired: 1 in]
            n135 = Add Array Elements(numeric array=w199) -> (sum=w198:i32)
          }
          frame #9 {
            "Notes" <- ""
          }
          frame #10 {
            n136 = Array Size(array=w225) -> (size(s)=w224:i32)
            n137 = Not Equal To 0?(x=w224) -> (x != 0?=w223:bool)
            n138 = case shown="True" w223 {
              tunnel: [enum16{"No Analogue data", "Take Analogue data"}."No Analogue data" ("Analogue data") enum16{"No Analogue data", "Take Analogue data"}."Take Analogue data" ("Analogue data")] -> w222
              frame False {
              }
              frame True {
              }
            }
            n139 = global write "Meas_global.vi" "Analogue data"(w222) -> ()
          }
          frame #11 {
            n140 = Index Array(array=w230, index=0) -> (element=w235:T23)
            n141 = Initialize Array(w235) -> (w233:T13)  [unwired: 1 out]
            n142 = Build Array (concatenate)(w230, w235) -> (w234:T13)
            n143 = for {
              N: w231 -> [_]
              tunnel: w234 -> [w243] mode=indexing
              shift-right: [w244] -> w229
              shift-left: w233 -> [w238]
              tunnel: Inst_type."Cross wire 2" ("Inst type") -> [w236]
              shift-right: [w242] -> _
              shift-left: _ -> [w241]
              tunnel: w234 -> [w240]
              n144 = Unbundle By Name(w243) -> ("Type"=w242:T3)
              n145 = Array Size(array=w238) -> (size(s)=w237:i32)
              n146 = Increment(x=w237) -> (x+1=w239:i32)
              n147 = case shown="\"Cross wire 1\"" w242 {
                tunnel: [w252 w272 w284] -> w244
                tunnel: w238 -> [w253 w274 w286]
                tunnel: w243 -> [w249 w275 w285]
                tunnel: w236 -> [w251 w279 _]
                tunnel: w241 -> [_ w278 _]
                tunnel: w240 -> [w256 _ _]
                tunnel: w239 -> [w255 _ _]
                frame "Cross wire 1" {
                  n148 = Index Array(array=w256, index=w255) -> (element=w250:T23)
                  n149 = Unbundle By Name(w250) -> ("Type"=w254:T3, "syncDelay"=w247:dbl, "Ch"=w246:i32, "Label"=w245:string)
                  n150 = Unbundle By Name(w249) -> ("Cal"=w248:path)
                  n151 = case shown="\"Generic Linear\", Default" w254 {
                    tunnel: w253 -> [w265 w271]
                    tunnel: [w264 w270] -> w252
                    tunnel: w251 -> [w258 w266]
                    tunnel: w248 -> [w263 w269]
                    tunnel: w249 -> [w261 w267]
                    tunnel: w247 -> [w260 _]
                    tunnel: w246 -> [w259 _]
                    tunnel: w245 -> [w257 _]
                    frame "Cross wire 2" {
                      n152 = Bundle By Name(cluster=w261, "Cal"=w263, "Type"=w258, "syncDelay"=w260, "Ch"=w259, "Label"=w257) -> (w262:T23)
                      n153 = Build Array (concatenate)(w265, w261, w262) -> (w264:T13)
                    }
                    frame "Generic Linear", Default {
                      n154 = Bundle By Name(cluster=w267, "Cal"=w269, "Type"=w266) -> (w268:T23)
                      n155 = Build Array (concatenate)(w271, w267, w268) -> (w270:T13)
                    }
                  }
                }
                frame "Cross wire 2" {
                  n156 = Decrement(x=w279) -> (x-1=w277:T3)
                  n157 = Equal?(x=w277, y=w278) -> (x = y?=w276:bool)
                  n158 = Bundle By Name(cluster=w275, "Type"=w277) -> (w273:T23)
                  n159 = case shown="False" w276 {
                    tunnel: w274 -> [w282 w283]
                    tunnel: w273 -> [w281 _]
                    tunnel: [w280 w283] -> w272
                    frame False {
                      n160 = Build Array (concatenate)(w282, w281) -> (w280:T13)
                    }
                    frame True {
                    }
                  }
                }
                frame "Generic Linear", Default {
                  n161 = Build Array (concatenate)(w286, w285) -> (w284:T13)
                }
              }
            }
          }
          frame #12 {
            n162 = Equal?(x=w288, y=Post_Process."Take New Data" ("Post Process")) -> (x = y?=w287:bool)
          }
          frame #13 {
          }
          frame #14 {
            n163 = And(x=w294, y=w292) -> (x .and. y?=w296:T4)
            n164 = case shown="True" w296 {
              tunnel: w293 -> [_ w306]
              tunnel: [FALSE w305] -> w297
              tunnel: [w298 w304] -> w295
              tunnel: w292 -> [w299 _]
              tunnel: w291 -> [_ w301]
              frame False {
                n165 = Not(x=w299) -> (.not. x?=w298:T4)
              }
              frame True {
                n166 = for {
                  shift-right: [w331] -> _
                  shift-left: string[] [] -> [w330]
                  tunnel: w306 -> [w329] mode=indexing
                  tunnel: [w321] -> w307 mode=indexing
                  shift-right: [w328] -> _
                  shift-left: path[] [] -> [w327]
                  tunnel: w301 -> [w309]
                  n167 = Unbundle By Name(w329) -> ("Type"=w326:T3, "Cal"=w317:path, "DAQ"=w310:string)
                  n168 = call "Full Channel ID.vi"("Cluster"=w329) -> ("String"=w314:string)
                  n169 = Equal?(x=w310, y=w309) -> (x = y?=w308:bool)
                  n170 = Search 1D Array(1D array=w330, element=w314) -> (index of element=w315:i32)  [unwired: 1 out]
                  n171 = Equal?(x=Inst_type."Fast FID" ("Inst type"), y=w326) -> (x = y?=w320:bool)
                  n172 = Less Than 0?(x=w315) -> (x < 0?=w313:bool)
                  n173 = Empty String/Path?(string/path=w314) -> (empty?=w312:bool)
                  n174 = Search 1D Array(1D array=w327, element=w317) -> (index of element=w324:i32)  [unwired: 1 out]
                  n175 = Compound Arithmetic op=OR(w312, w313, w308) -> (w311:bool)
                  n176 = Empty String/Path?(string/path=w317) -> (empty?=w316:bool)
                  n177 = Greater Or Equal To 0?(x=w324) -> (x >= 0?=w319:bool)
                  n178 = case shown="False" w311 {
                    tunnel: w314 -> [w342 _]
                    tunnel: [w338 FALSE ("true")] -> w323
                    frame False {
                      n179 = Format Into String(format string="The Channel %s appears more than once", w342) -> (resulting string=w340:string)  [unwired: 2 in, 1 out]
                      n180 = One Button Dialog(message=w340, button name ("OK")="Ok") -> (true=w338:bool)
                    }
                    frame True {
                    }
                  }
                  n181 = Compound Arithmetic op=AND(w319, w320, invert w316) -> (w318:bool)
                  n182 = case shown="True" w318 {
                    tunnel: [w333 FALSE ("true")] -> w322
                    tunnel: w317 -> [w332 _]
                    frame True {
                      n183 = Format Into String(format string="Calibration file %s is used more than once.", w332) -> (resulting string=w335:string)  [unwired: 2 in, 1 out]
                      n184 = One Button Dialog(message=w335, button name ("OK")="Ok") -> (true=w333:bool)
                    }
                    frame False {
                    }
                  }
                  n185 = Build Array (concatenate)(w330, w314) -> (w331:string[])
                  n186 = Build Array (concatenate)(w327, w317) -> (w328:path[])
                  n187 = Or(x=w323, y=w322) -> (x .or. y?=w321:bool)
                }
                n188 = Or Array Elements(Boolean array=w307) -> (logical OR=w304:bool)
                n189 = Not(x=w304) -> (.not. x?=w305:bool)
              }
            }
          }
          frame #15 {
            n190 = case shown="\"Take New Data\"" w344 {
              tunnel: w346 -> [w348 w382]
              tunnel: [w347 w382] -> w345
              frame "Take New Data" {
                n191 = call "Current_Calib_Filenames.vi"("Mode"=App_Global."Read Global") -> ("Calib Filename Out"=w349:path[], "Channel ID Output"=w350:string[])  [unwired: 2 in, 1 out]
                n192 = for {
                  tunnel: w348 -> [w360] mode=indexing
                  tunnel: w350 -> [w366]
                  tunnel: w349 -> [w365]
                  tunnel: [w357] -> w347 mode=indexing
                  n193 = Unbundle By Name(w360) -> ("Type"=w356:T3, "calType"=w354:T11)
                  n194 = call "Full Channel ID.vi"("Cluster"=w360) -> ("String"=w359:string)
                  n195 = Equal?(x=w354, y=calType."Latest" ("calType")) -> (x = y?=w352:bool)
                  n196 = Not Equal?(x=w356, y=Inst_type."Cross wire 2" ("Inst type")) -> (x != y?=w355:bool)
                  n197 = Not Equal?(x=Inst_type."Raw voltage" ("Inst type"), y=w356) -> (x != y?=w361:bool)
                  n198 = Compound Arithmetic op=AND(w352, w355) -> (w363:bool)
                  n199 = case shown="True" w363 {
                    tunnel: w366 -> [_ w381]
                    tunnel: w359 -> [_ w380]
                    tunnel: w365 -> [_ w378]
                    tunnel: w360 -> [w371 w377]
                    tunnel: [w371 w376] -> w358
                    tunnel: w361 -> [_ w373]
                    frame False {
                    }
                    frame True {
                      n200 = Search 1D Array(1D array=w381, element=w380) -> (index of element=w379:i32)  [unwired: 1 out]
                      n201 = Index Array(array=w378, index=w379) -> (element=w374:path)
                      n202 = Select(t=w374, s=w373, f=path "") -> (s? t:f=w375:path)
                      n203 = Bundle By Name(cluster=w377, "Cal"=w375) -> (w376:T23)
                    }
                  }
                  n204 = in-place {
                    n205 = in-place-cluster #1(w358) -> ("Fs"=w368:dbl)
                    n206 = Equal To 0?(x=w368) -> (x = 0?=w370:bool)
                    n207 = Select(t=200.0, s=w370, f=w368) -> (s? t:f=w367:dbl)
                    n208 = in-place-cluster #1("Fs"=w367) -> (w357:T23)
                  }
                }
              }
              frame "Post Process Raw Data File" {
              }
            }
          }
          frame #16 {
            n209 = case shown="True" w385 {
              tunnel: w384 -> [w387 w390]
              tunnel: [w387 w389] -> w383
              tunnel: w386 -> [_ w388]
              frame False {
              }
              frame True {
                n210 = case shown="\"Run Program\", Default" w388 {
                  tunnel: w390 -> [w392 w402]
                  tunnel: [w391 w402] -> w389
                  frame "Run Program", Default {
                    n211 = for {
                      tunnel: w392 -> [w398] mode=indexing
                      tunnel: [w399] -> w391 mode=indexing
                      n212 = Unbundle By Name(w398) -> ("Cal"=w401:path, "calType"=w397:T11, "Type"=w400:T3)
                      n213 = call "Full Channel ID.vi"("Cluster"=w398) -> ("String"=w395:string)
                      n214 = Equal?(x=w397, y=calType."Latest" ("calType")) -> (x = y?=w393:bool)
                      n215 = call "Find_calibration_file.vi"("Inst type"=w400, "Channel ID"=w395, "Use Latest Calib"=w393, "filename"=w401) -> ("filename out"=w396:path)
                      n216 = Bundle By Name(cluster=w398, "Cal"=w396) -> (w399:T23)
                    }
                  }
                  frame "Setup Front Panel" {
                  }
                }
              }
            }
          }
          frame #17 {
            n217 = global read "Meas_global.vi" "Acquisition_Plug_Ins to Run"() -> (w408:string[])
            n218 = Equal?(x=w406, y=w408) -> (x = y?=w407:bool[])
            n219 = Or Array Elements(Boolean array=w407) -> (logical OR=w405:bool)
            n220 = Equal?(x=w409, y=Post_Process."Take New Data" ("Post Process")) -> (x = y?=w404:bool)
            n221 = And(x=w404, y=w405) -> (x .and. y?=w403:bool)
          }
          frame #18 {
            n222 = case shown="True" w413 {
              tunnel: w411 -> [w415 w422]
              tunnel: w414 -> [_ w421]
              tunnel: [w415 w418] -> w412
              frame False {
              }
              frame True {
                n223 = call "Get_ADAM_Ch_names_client.vi"("Channel names set"=Channel_names."Active + Off") -> ("Ch names"=w419:string[])
                n224 = call "Get_ADAM_Ch_names_client.vi"("Channel names set"=Channel_names."Active Only") -> ("Ch names"=w416:string[])
                n225 = for {
                  tunnel: w422 -> [w426] mode=indexing
                  tunnel: w421 -> [w430]
                  tunnel: w419 -> [w429]
                  tunnel: [w425] -> w418 mode=indexing
                  tunnel: w416 -> [w424]
                  i -> [w427]
                  n226 = Unbundle By Name(w426) -> ("Label"=w423:string, "DAQ"=w431:string)
                  n227 = Equal?(x=w431, y=w430) -> (x = y?=w428:bool)
                  n228 = case shown="True" w428 {
                    tunnel: w429 -> [_ w441]
                    tunnel: w423 -> [_ w437]
                    tunnel: w427 -> [_ w438]
                    tunnel: w426 -> [w432 w439]
                    tunnel: [w432 w436] -> w425
                    tunnel: w424 -> [_ w435]
                    frame False {
                    }
                    frame True {
                      n229 = Search 1D Array(1D array=w441, element=w437) -> (index of element=w440:i32)  [unwired: 1 in]
                      n230 = case shown="-1" w440 {
                        tunnel: w441 -> [_ w451]
                        tunnel: w438 -> [_ w449]
                        tunnel: [w445 w446] -> w433
                        tunnel: w437 -> [w445 _]
                        frame Default {
                        }
                        frame -1 {
                          n231 = Format Into String(format string="Please select the required ADAM channel for index %d from the Server" ("Message"), w449) -> (resulting string=w448:string)  [unwired: 2 in, 1 out]
                          n232 = call "Select_Strings.vi"("Available Ch names"=w451, "Message"=w448, "Selector mode"=T20."One") -> ("Selected Channel Names"=w447:string[])  [unwired: 2 in, 3 out]
                          n233 = Index Array(array=w447) -> (element=w446:string)  [unwired: 1 in]
                        }
                      }
                      n234 = Search 1D Array(1D array=w435, element=w433) -> (index of element=w434:i32)  [unwired: 1 in]
                      n235 = case shown="-1" w434 {
                        tunnel: w433 -> [_ w444]
                        frame Default {
                        }
                        frame -1 {
                          n236 = call "Ch_Active_Control_Client.vi"("Match"=w444, "Activate Channels?"=TRUE, "Control on"=Channel_State_Control."Channel Name") -> ()  [unwired: 2 out]
                        }
                      }
                      n237 = Bundle By Name(cluster=w439, "Label"=w433, "Ch"=w438) -> (w436:T23)
                    }
                  }
                }
              }
            }
          }
          frame #19 {
            (unwired) "Dynamically Added" ("Port")
            n238 = global read "Meas_global.vi" "Dynamically Added"() -> (w456:T21[])
            n239 = Build Array (concatenate)(w455, w456) -> (w454:T21[])
            n240 = for {
              shift-right: [w467] -> _
              shift-left: string[] [] -> [w468]
              tunnel: [w464] -> w458 mode=indexing
              tunnel: w454 -> [w466] mode=indexing
              tunnel: [w463] -> w457 mode=indexing
              tunnel: [w460] -> w453 mode=indexing
              # "#ToDo Maybe make this more generic..?"
              n241 = Unbundle By Name(w466) -> ("Type"=w469:T3, "Port"=w462:T10)
              n242 = case shown="\"Cross wire 1\"" w469 {
                tunnel: [w480 w484 w487 w491 w495 w499 w503 "XW" w510 w514 w519 w522 w526] -> w464
                tunnel: ["U" "P" "U" "U" "U" "U" "U" "W" "U" "V" "C" "T" "T"] -> w470
                tunnel: w468 -> [w481 w485 w489 w493 w497 w501 w505 w507 w512 w516 w520 w524 w528]
                tunnel: [w479 w483 w488 w492 w496 w500 w504 w507 w511 w515 w518 w523 w527] -> w467
                frame "Propeller anemometer" {
                  w480 = "Prop"
                  n243 = Build Array (concatenate)(w481, w480) -> (w479:string[])
                }
                frame "Pressure Transducer" {
                  w484 = "Mano"
                  n244 = Build Array (concatenate)(w485, w484) -> (w483:string[])
                }
                frame "Raw voltage" {
                  w487 = "RV"
                  n245 = Build Array (concatenate)(w489, w487) -> (w488:string[])
                }
                frame "Raw with zero offsetting" {
                  w491 = "RZ"
                  n246 = Build Array (concatenate)(w493, w491) -> (w492:string[])
                }
                frame "Pitot-static tube" {
                  w495 = "Pitot"
                  n247 = Build Array (concatenate)(w497, w495) -> (w496:string[])
                }
                frame "Hot wire" {
                  w499 = "HW"
                  n248 = Build Array (concatenate)(w501, w499) -> (w500:string[])
                }
                frame "Cross wire 1" {
                  w503 = "XW"
                  n249 = Build Array (concatenate)(w505, w503) -> (w504:string[])
                }
                frame "Cross wire 2" {
                }
                frame "Generic Linear", Default {
                  w510 = "Gen"
                  n250 = Build Array (concatenate)(w512, w510) -> (w511:string[])
                }
                frame "Microphone" {
                  w514 = "Mic"
                  n251 = Build Array (concatenate)(w516, w514) -> (w515:string[])
                }
                frame "Fast FID" {
                  w519 = "FF"
                  n252 = Build Array (concatenate)(w520, w519) -> (w518:string[])
                }
                frame "Thermocouple" {
                  w522 = "T"
                  n253 = Build Array (concatenate)(w524, w522) -> (w523:string[])
                }
                frame "Cold wire" {
                  w526 = "CW"
                  n254 = Build Array (concatenate)(w528, w526) -> (w527:string[])
                }
              }
              n255 = call "Analyse_string_array.vi"("String array"=w467) -> ("Unique strings"=w474:string[], "Frequency"=w472:i32[])  [unwired: 1 out]
              n256 = Search 1D Array(1D array=w474, element=w464) -> (index of element=w473:i32)  [unwired: 1 out]
              n257 = Index Array(array=w472, index=w473) -> (element=w465:i32)
              n258 = Number To Decimal String(number=w465) -> (decimal integer string=w463:string)  [unwired: 1 out]
              n259 = Concatenate Strings(w463, w464, ":", w470) -> (w461:string)
              n260 = case shown="\"False\", Default" w462 {
                tunnel: w461 -> [w475 w477]
                tunnel: [w475 w476] -> w460
                frame "False", Default {
                }
                frame "Dynamically Added" {
                  n261 = Concatenate Strings(w477, " Derived" ("string")) -> (w476:string)
                }
              }
            }
          }
          frame #20 {
            n262 = for {
              tunnel: w530 -> [w556] mode=indexing
              tunnel: w536 -> [w564] mode=indexing
              tunnel: [w565] -> w533 mode=indexing
              tunnel: w535 -> [w557] mode=indexing
              tunnel: w534 -> [w561] mode=indexing
              tunnel: w532 -> [_]
              tunnel: w531 -> [w546]
              w548 = string[] [] ("Metadata Ch Names")
              n263 = Unbundle By Name(w556) -> ("Label"=w540:string, "Port"=w549:T10, "calType"=w543:T11, "syncDelay"=w554:dbl, "Ch"=w550:i32, "Type"=w559:T3, "DAQ"=w539:string, "Fs"=w551:dbl, "chState"=w537:T9)  [unwired: 1 out]
              n264 = Empty String/Path?(string/path=w540) -> (empty?=w562:bool)
              n265 = Select(t=w561, s=w562, f=w540) -> (s? t:f=w560:string)
              n266 = Format Into String(format string="%s (%s)" ("Format String"), w564, w560) -> (resulting string=w547:string)  [unwired: 2 in, 1 out]
              n267 = call <vilib>:"Trim Whitespace.vi"("string"=w540) -> ("trimmed string"=w545:string)  [unwired: 1 in]
              n268 = Divide(x=w554, y=1000.0) -> (x/y=w553:dbl)
              n269 = Format Into String(format string="Ch %d" ("Format String"), w550) -> (resulting string=w552:string)  [unwired: 2 in, 1 out]
              n270 = Equal?(x=w543, y=calType."Latest" ("calType")) -> (x = y?=w542:bool)
              n271 = Bundle By Name(cluster=w546, "Label"=w545, "Metadata Ch Names"=w548, "Metadata Ch Values"=w548, "Port"=w549, "Use Latest Calib"=w542, "Extra Info"=w552, "Device"=w539, "Inst type"=w559, "Inst name"=w547, "Symbol"="", "Code name"=w557, "Inst Array"=Instrument_Array."Analogue", "Sync Delay Time (s)"=w553, "Req Sample Rate Hz"=w551, "Ch No"=w550, "chState"=w537) -> (w565:T7)
            }
          }
          frame #21 {
            n272 = Not Equal?(x=w566, y=w567) -> (x != y?=w568:bool)
            n273 = case shown="True" w568 {
              tunnel: w567 -> [_ w569]
              frame False {
              }
              frame True {
                n274 = local write "Ch & spans choices"(w569) -> ()
              }
            }
          }
          frame #22 {
          }
          frame #23 {
            n275 = case shown="\"No LDA data\"" "LDA data" {
              tunnel: w570 -> [_ w577]
              tunnel: [w574 w578] -> w572
              frame "No LDA data" {
                w574 = u8 2  # Disabled
                n276 = local write "Use  Analogue channel to software sync with LDA"(FALSE ("Synchronise Analogue channels with LDA")) -> ()
              }
              frame "Take LDA data" {
                n277 = Array Size(array=w577) -> (size(s)=w576:i32)
                n278 = Not Equal To 0?(x=w576) -> (x != 0?=w575:bool)
                n279 = case shown="True" w575 {
                  selector: w575 -> [w579 _]
                  tunnel: [u8 2 ("Disabled") u8 0 ("Disabled")] -> w578
                  frame False {
                    n280 = local write "Use  Analogue channel to software sync with LDA"(w579) -> ()
                  }
                  frame True {
                  }
                }
              }
            }
            n281 = property on="Use  Analogue channel to software sync with LDA" class="Bool (strict)"("Disabled"=w572) -> ()  [unwired: 2 in, 2 out]
          }
          frame #24 {
            n282 = local read "XW Present?"() -> (w584:bool)
            n283 = case shown="False" w584 {
              tunnel: [w585 "Cross wire"] -> w583
              frame False {
                w585 = T6."2nd component as calculated"  # Cross wire/LDA
              }
              frame True {
              }
            }
            n284 = property on="Cross wire/LDA" class="Enum (strict)"("Visible"=w584) -> ()  [unwired: 2 in, 2 out]
            n285 = global write "Meas_global.vi" "Cross wire + or -ve"(w583) -> ()
            n286 = Wait (ms)(milliseconds to wait=u32 100) -> ()  [unwired: 1 out]
          }
          frame #25 {
            n287 = local read "Use  Analogue channel to software sync with LDA"() -> (w592:bool)
            n288 = And(x=w594, y=w595) -> (x .and. y?=w593:T4)
            n289 = while {
              shift-left: _ -> [w619]
              shift-right: [w620] -> w589
              tunnel: [w621] -> w591
              stop <- FALSE continue-if-true
              n290 = local read "Setup filename selector"() -> (w620:u16)
              n291 = Not Equal?(x=w620, y=w619) -> (x != y?=w621:bool)
            }
            n292 = case shown="True" w592 {
              tunnel: w587 -> [_ w605]
              tunnel: w593 -> [_ w604]
              frame False {
              }
              frame True {
                n293 = case shown="True" w604 {
                  tunnel: w605 -> [_ w608]
                  frame False {
                  }
                  frame True {
                    n294 = for {
                      tunnel: w608 -> [w617] mode=indexing
                      tunnel: [w610] -> w607 mode=indexing
                      n295 = Unbundle By Name(w617) -> ("Type"=w616:T3, "Label"=w614:string)
                      n296 = Equal?(x=w614, y="Sync") -> (x = y?=w612:bool)
                      n297 = Equal?(x=Inst_type."Raw voltage" ("Inst type"), y=w616) -> (x = y?=w611:bool)
                      n298 = And(x=w611, y=w612) -> (x .and. y?=w610:bool)
                    }
                    n299 = Or Array Elements(Boolean array=w607) -> (logical OR=w606:bool)
                    n300 = case shown="False" w606 {
                      frame False {
                        n301 = One Button Dialog(message="To Perform LDA Sync you must provide a Raw voltage channel having the symbol \"Sync\"") -> ()  [unwired: 2 out]
                      }
                      frame True {
                      }
                    }
                  }
                }
              }
            }
            n302 = case shown="True" w591 {
              tunnel: [FALSE ("exists?") w603] -> w590
              tunnel: w589 -> [_ w601]
              frame False {
              }
              frame True {
                n303 = local read "Setup Paths"() -> (w602:string[])
                n304 = Index Array(array=w602, index=w601) -> (element=w599:string)
                n305 = call "Setup_Filepath.vi"("Setup File Type"=Setup_Filetype."Measurement Setups", "Filename in"=w599) -> ("Filename Out"=w598:path)  [unwired: 1 out]
                n306 = call "Does_file_exist_(simple).vi"("Pathname"=w598) -> ("exists?"=w603:bool)
              }
            }
            n307 = local write "Read Setup File?"(w590) -> ()
            n308 = global write "Meas_global.vi" "Aborted Setup"("stop") -> ()
            n309 = Current VI's Path() -> (path=w596:path)
            n310 = call "Close_Panel_and_Abort.vi"("Vi path"=w596, "stop"="stop") -> ()  [unwired: 1 out]
          }
        }
      }
    }
    frame #5 {
      n311 = local read "LDA data"() -> (w624:enum16{"No LDA data", "Take LDA data"})
      n312 = case shown="\"Take LDA data\"" w624 {
        tunnel: [FALSE ("Synchronise Analogue channels with LDA") "Use  Analogue channel to software sync with LDA"] -> w623
        tunnel: [0 ("Number of LDA Chs") "Number of LDA Chs"] -> w622
        frame "No LDA data" {
        }
        frame "Take LDA data" {
        }
      }
      n313 = global write "Meas_global.vi" "LDA data"(w624) -> ()
      n314 = global write "LDA_global.vi" "Number of LDA Chs"(w622) -> ()
      n315 = global write "Meas_global.vi" "Use  Analogue channel to software sync with LDA"(w623) -> ()
    }
    frame #6 {
      n316 = global read "Meas_global.vi" "Pre Setup String"() -> (w629:string)
      n317 = stacked-sequence {
        seq-local: [_ w659 _ _ _ _] -> [_ _ _ w708 _ _]
        seq-local: [_ _ w678 _ _ _] -> [_ _ _ w707 _ _]
        seq-local: [w635 _ _ _ _ _] -> [_ _ _ w701 _ _]
        seq-local: [_ _ _ w695 _ _] -> [_ _ _ _ _ w747]
        seq-local: [_ _ _ _ w713 _] -> [_ _ _ _ _ w748]
        tunnel: w631 -> [w634 _ _ w702 _ _]
        tunnel: w630 -> [w633 _ _ _ _ _]
        tunnel: w629 -> [w632 _ _ w696 _ w746]
        frame #0 {
          n318 = local read "PWA Data"() -> (w636:T2)
          n319 = case shown="\"One Ch PWA\"" w636 {
            tunnel: ["" w646] -> w635
            tunnel: w634 -> [_ w645]
            tunnel: w633 -> [_ w641]
            tunnel: w632 -> [_ w638]
            frame "No PWA Data" {
            }
            frame "One Ch PWA" {
              n320 = Not Equal?(x="Calib_Setup.xls", y=w641) -> (x != y?=w640:bool)
              n321 = case shown="\"Setup Front Panel\"" w645 {
                tunnel: [w649 w652 w655 w658] -> w644
                tunnel: [w648 w651 w654 w657] -> w643
                tunnel: [w647 w650 w653 w656] -> w639
                tunnel: w640 -> [w647 w650 w653 _]
                frame "Show Setup" {
                  w649 = TRUE  # Show Panel?
                  w648 = T4 FALSE  # OK
                }
                frame "Run Program" {
                  w652 = FALSE  # Show Panel?
                  w651 = T4 TRUE  # OK
                }
                frame "Save Current Setup" {
                  w655 = FALSE  # Show Panel?
                  w654 = T4 TRUE  # OK
                }
                frame "Setup Front Panel" {
                  w656 = FALSE  # Check Calib file?
                  w658 = FALSE  # Show Panel?
                  w657 = T4 TRUE  # OK
                }
              }
              n322 = call "PWA_Setup_Panel.vi"("Show Panel?"=w644, "Check Calib file?"=w639, "OK"=w643, "Incoming Setup String"=w638) -> ("Outgoing Setup String"=w646:string)  [unwired: 3 out]
            }
          }
        }
        frame #1 {
          n323 = local read "DAQ Tigger Control?"() -> (w663:bool)
          n324 = Select(t="Port", s=w663, f="") -> (s? t:f=w660:refnum<visa-resource-name>)
          n325 = call "Characters_to_string.vi"("Characters to write"=w660, "Label for characters"="DAQ External Trigger Port") -> ("Output string"=w659:string)  [unwired: 1 in]
        }
        frame #2 {
          n326 = global read "Preference_global.vi" "Rig Setup"() -> (w667:string)
          n327 = local read "Cross wire"() -> (w681:T6)
          n328 = case shown="\"Trigger Every Sample\"" "Trigger mode" {
            tunnel: ["Free Running" "Trigger Every Block" "Trigger Every Sample" "Start on Trigger"] -> w676
            frame "Free Running" {
            }
            frame "Trigger Every Block" {
            }
            frame "Trigger Every Sample" {
            }
            frame "Start on Trigger" {
            }
          }
          n329 = global write "Meas_global.vi" "Trigger mode"("Trigger mode") -> ()
          n330 = Match Pattern(string=w667, regular expression="-") -> (before substring=w666:string)  [unwired: 4 out]
          n331 = property on="PWA Data" class="Enum (strict)"() -> ("Strings []"=w672:string[])  [unwired: 2 in, 2 out]
          n332 = Equal?(x=T6."2nd component multipled by -1" ("Cross wire/LDA"), y=w681) -> (x = y?=w680:bool)
          n333 = case shown="\"EnFlo_Tunnel\"" w666 {
            tunnel: ["" w688] -> w665
            frame "False", Default {
            }
            frame "EnFlo_Tunnel" {
              n334 = call "Characters_to_string.vi"("Characters to write"="FALSE", "Label for characters"="Show_all_EnFlo_Tunnel_Columns") -> ("Output string"=w688:string)  [unwired: 1 in]
            }
          }
          n335 = global write "Meas_global.vi" "PWA Data"("PWA Data") -> ()
          n336 = Index Array(array=w672, index="PWA Data") -> (element=w671:string)
          n337 = Select(t="TRUE", s=w680, f="FALSE") -> (s? t:f=w683:string)
          n338 = call "Characters_to_string.vi"("Characters to write"=w671, "Label for characters"="Pulsed_Wire_Data" ("Variable name")) -> ("Output string"=w670:string)  [unwired: 1 in]
          n339 = call "Characters_to_string.vi"("Characters to write"=w683, "Label for characters"="Invert Second Component") -> ("Output string"=w679:string)  [unwired: 1 in]
          n340 = call "Characters_to_string.vi"("Characters to write"=w676, "Label for characters"="Trigger mode") -> ("Output string"=w674:string)  [unwired: 1 in]
          n341 = Concatenate Strings(w674, w670, w679, w665) -> (w678:string)
        }
        frame #3 {
          w700 = "Setup Info for Plug_Ins" ("File Label")
          w703 = FALSE  # Show Panel?
          n342 = call "Choose_Plug_In_to_Run.vi"("setup"=w702, "Show Panel?"=w703, "Setup String In"=w696) -> ("Setup String Out"=w704:string)  [unwired: 1 out]
          n343 = call "Get_string_subset.vi"("String to split"=w696, "File Label"=w700) -> ("Output string"=w698:string)  [unwired: 2 in, 1 out]
          n344 = Empty String/Path?(string/path=w698) -> (empty?=w697:bool)
          n345 = call "Date_and_Time_to_string.vi"() -> ("Date and time (spreadsheet)"=w706:string)  [unwired: 4 in, 1 out]
          n346 = case shown="False" w697 {
            tunnel: w700 -> [w711 _]
            tunnel: [w710 ""] -> w699
            tunnel: w698 -> [w709 _]
            frame False {
              n347 = call "Add_label_to_string.vi"("String to write"=w709, "File Label"=w711) -> ("Output string"=w710:string)
            }
            frame True {
            }
          }
          n348 = global read "Meas_global.vi" "New Setup String"() -> (w705:string)
          n349 = Concatenate Strings(w705, w701, w704, w706, w708, w707, w699) -> (w695:string)
        }
        frame #4 {
          n350 = call "Plug_in_Directories.vi"() -> ("Initial"=w714:path, "Pre_Analysis_Plugins"=w715:path, "Per Block"=w716:path, "Final"=w717:path)  [unwired: 2 in, 1 out]
          n351 = Strip Path(path=w716) -> (name=w722:string)  [unwired: 1 out]
          n352 = Strip Path(path=w717) -> (name=w723:string)  [unwired: 1 out]
          n353 = Strip Path(path=w714) -> (name=w718:string)  [unwired: 1 out]
          n354 = Strip Path(path=w715) -> (name=w728:string)  [unwired: 1 out]
          n355 = global read "Dynamic_call_global.ph.vi" "Pre_Analysis Plug Ins"() -> (w727:string[])
          n356 = global read "Dynamic_call_global.ph.vi" "Initial Plug Ins"() -> (w719:string[])
          n357 = global read "Dynamic_call_global.ph.vi" "Per Block Plug Ins"() -> (w721:string[])
          n358 = global read "Dynamic_call_global.ph.vi" "Final Plug Ins"() -> (w720:string[])
          n359 = for {
            tunnel: w718 -> [w744]
            tunnel: w719 -> [w743] mode=indexing
            tunnel: [w742] -> w724 mode=indexing
            n360 = Concatenate Strings(w744, "__" ("string"), w743) -> (w742:string)
          }
          n361 = for {
            tunnel: w728 -> [w732]
            tunnel: w727 -> [w731] mode=indexing
            tunnel: [w730] -> w729 mode=indexing
            n362 = Concatenate Strings(w732, "__" ("string"), w731) -> (w730:string)
          }
          n363 = for {
            tunnel: w723 -> [w736]
            tunnel: w720 -> [w735] mode=indexing
            tunnel: [w734] -> w726 mode=indexing
            n364 = Concatenate Strings(w736, "__" ("string"), w735) -> (w734:string)
          }
          n365 = for {
            tunnel: w722 -> [w740]
            tunnel: w721 -> [w739] mode=indexing
            tunnel: [w738] -> w725 mode=indexing
            n366 = Concatenate Strings(w740, "__" ("string"), w739) -> (w738:string)
          }
          n367 = Build Array (concatenate)(w724, w729, w725, w726) -> (w713:string[])
        }
        frame #5 {
          n368 = for {
            shift-right: [w753] -> w751
            shift-left: "" -> [w754]
            tunnel: w748 -> [w755] mode=indexing
            tunnel: w746 -> [w752]
            n369 = call "Get_string_subset.vi"("String to split"=w752, "File Label"=w755) -> ("Output string"=w757:string)  [unwired: 2 in, 1 out]
            n370 = Empty String/Path?(string/path=w757) -> (empty?=w756:bool)
            n371 = case shown="False" w756 {
              tunnel: w755 -> [w762 _]
              tunnel: [w758 w763] -> w753
              tunnel: w757 -> [w761 _]
              tunnel: w754 -> [w760 w763]
              frame False {
                n372 = call "Add_label_to_string.vi"("String to write"=w761, "File Label"=w762) -> ("Output string"=w759:string)
                n373 = Concatenate Strings(w760, w759) -> (w758:string)
              }
              frame True {
              }
            }
          }
          n374 = Concatenate Strings(w747, w751) -> (w750:string)
          n375 = global write "Meas_global.vi" "New Setup String"(w750) -> ()
        }
      }
    }
    frame #7 {
      n376 = case shown="\"Take New Data\"" w766 {
        tunnel: w765 -> [w773 w814]
        tunnel: [w768 w808] -> w764
        frame "Take New Data" {
          n377 = for {
            tunnel: w773 -> [w776] mode=indexing
            shift-right: [w781] -> w771
            shift-left: string[] [] -> [w782]
            shift-right: [w779] -> w770
            shift-left: path[] [] -> [w780]
            tunnel: [w774] -> w768 mode=indexing
            n378 = Unbundle By Name(w776) -> ("calType"=w778:T11, "DAQ"=w783:string, "Cal"=w777:path)
            n379 = call "Full Channel ID.vi"("Cluster"=w776) -> ("String"=w775:string)
            n380 = case shown="\"Propeller anemometer\", Default" w783 {
              tunnel: w782 -> [w793 w804 w807]
              tunnel: w775 -> [w792 _ _]
              tunnel: [w791 w804 w807] -> w781
              tunnel: w780 -> [w790 w803 w806]
              tunnel: w777 -> [w785 w802 w805]
              tunnel: [w789 w803 w806] -> w779
              tunnel: w778 -> [w788 _ _]
              tunnel: [w784 w802 w805] -> w774
              frame "Propeller anemometer", Default {
                n381 = case shown="\"Latest\"" w788 {
                  tunnel: w793 -> [w799 w801]
                  tunnel: w792 -> [w798 _]
                  tunnel: [w797 w801] -> w791
                  tunnel: w790 -> [w796 w800]
                  tunnel: w785 -> [w795 _]
                  tunnel: [w794 w800] -> w789
                  frame "Latest" {
                    n382 = Build Array (concatenate)(w799, w798) -> (w797:string[])
                    n383 = Build Array (concatenate)(w796, w795) -> (w794:path[])
                  }
                  frame "Fixed" {
                  }
                }
                n384 = call "Current_Filepath.vi"("Short_Name"="Cal" ("Data Type"), "Filename in"=w785, "Data Type"="Calibrations") -> ("Filename Out"=w784:path)  [unwired: 1 in, 1 out]
              }
              frame "Raw voltage" {
              }
              frame "Raw with zero offsetting" {
              }
            }
          }
          n385 = call "Current_Calib_Filenames.vi"("Calib Filename"=w770, "Channel ID input"=w771, "Mode"=App_Global."Write to Global") -> ()  [unwired: 3 out]
        }
        frame "Post Process Raw Data File" {
          n386 = for {
            tunnel: w814 -> [w820] mode=indexing
            tunnel: [w819] -> w808 mode=indexing
            n387 = Unbundle By Name(w820) -> ("Cal"=w819:path)
          }
          n388 = global read "Meas_global.vi" "Pre Setup String"() -> (w813:string)
          n389 = call "Get_Characters_from_string.vi"("Input string"=w813, "Variable name"="Skip_Block_Numbers_(eg 1;2;5;12)") -> ("Status"=w811:enum16{"Char in string", "Char not in string"}, "Value"=w810:string)  [unwired: 1 in]
          n390 = case shown="\"Char in string\"" w811 {
            tunnel: w810 -> [w817 _]
            tunnel: [w815 i32[] []] -> w809
            frame "Char in string" {
              n391 = call "Get_array_values_fr_String.vi"("String Value"=w817) -> ("Numeric Array"=w816:dbl[])  [unwired: 1 out]
              n392 = To Long Integer(number=w816) -> (32bit integer=w815:i32[])
            }
            frame "Char not in string" {
            }
          }
          n393 = global write "Meas_global.vi" "Blocks to Skip"(w809) -> ()
        }
      }
    }
    frame #8 {
      n394 = global read "LDA_global.vi" "Number of LDA Chs"() -> (w821:i32)
      n395 = global read "LDA_global.vi" "LDA Channels"() -> (w825:T22[])
      n396 = global read "Meas_global.vi" "Pre Setup String"() -> (w822:string)
      n397 = for {
        N: w821 -> [_]
        tunnel: w826 -> [w851]
        tunnel: w825 -> [w850] mode=indexing
        tunnel: " Sync Delay (ms)" -> [w832]
        tunnel: [w830] -> w823 mode=indexing
        tunnel: w822 -> [w829]
        i -> [w838]
        n398 = Unbundle By Name(w850) -> ("BSA IP"=w827:string, "Vel Comp"=w846:string, "COLOUR"=w842:u32, "Req Sampling Rate Hz"=w839:dbl, "Sync Delay (s)"=w828:dbl)
        n399 = Increment(x=w838) -> (x+1=w844:i32)
        n400 = Format Into String(format string="%dLDA:U" ("Bundle Element"), w844) -> (resulting string=w833:string)  [unwired: 2 in, 1 out]
        n401 = Format Into String(format string="LDA (%s)" ("Format String"), w846) -> (resulting string=w843:string)  [unwired: 2 in, 1 out]
        n402 = Concatenate Strings(w833, w832) -> (w834:string)
        n403 = call "Get_value_from_string.vi"("Input string"=w829, "Variable name"=w834) -> ("Status"=w836:enum16{"Char in string", "Char not in string"}, "Value"=w835:dbl)  [unwired: 1 in]
        n404 = case shown="\"Char not in string\"" w836 {
          tunnel: w835 -> [w857 _]
          tunnel: [w852 w858] -> w831
          tunnel: w828 -> [_ w858]
          frame "Char in string" {
            n405 = Divide(x=w857, y=1000.0) -> (x/y=w854:dbl)
            n406 = Not A Number/Path/Refnum?(number/path/refnum=w854) -> (NaN/Path/Refnum?=w855:bool)
            n407 = Select(t=0.0, s=w855, f=w854) -> (s? t:f=w852:dbl)
          }
          frame "Char not in string" {
          }
        }
        n408 = Bundle By Name(cluster=w851, "Port"=w827, "Stats"=enum16{"None", "Basic", "Full"}."Full", "Inst type"=Inst_type."LDA Vel", "Label"=w846, "Code name"=w833, "Inst name"=w843, "Colour"=w842, "Extra Info"="", "Inst Array"=Instrument_Array."LDA" ("Instrument Array"), "Req Sample Rate Hz"=w839, "Ch No"=w838, "Device"="LDA_IP.vi" ("Device ID"), "Sync Delay Time (s)"=w831) -> (w830:T7)
      }
    }
    frame #9 {
      n409 = global read "Meas_global.vi" "Pre Setup String"() -> (w867:string)
      n410 = for {
        tunnel: [w886] -> w866 mode=indexing
        tunnel: w860 -> [w884] mode=indexing
        tunnel: w861 -> [w879] mode=indexing
        tunnel: w867 -> [w885]
        n411 = Unbundle By Name(w884) -> ("Code name"=w883:string)
        n412 = Concatenate Strings(w883, "_Av_SamplingRate" ("string")) -> (w881:string)
        n413 = call "Get_value_from_string.vi"("Input string"=w885, "Variable name"=w881) -> ("Value"=w880:dbl)  [unwired: 1 in, 1 out]
        n414 = Bundle By Name(cluster=w884, "Calib File"=w879, "Av Sampling Rate"=w880) -> (w886:T7)
      }
      n415 = global read "Meas_global.vi" "Dynamically Added"() -> (w863:T21[])
      n416 = Array Size(array=w863) -> (size(s)=w859:i32)
      n417 = Greater Than 0?(x=w859) -> (x > 0?=w862:bool)
      n418 = case shown="True" w862 {
        tunnel: w866 -> [w870 w878]
        tunnel: [w869 w877] -> w865
        tunnel: w864 -> [w868 w876]
        tunnel: w861 -> [_ w875]
        tunnel: w860 -> [_ w874]
        tunnel: w859 -> [_ w872]
        frame False {
          n419 = Build Array (concatenate)(w868, w870) -> (w869:T7[])
        }
        frame True {
          n420 = Array Size(array=w875) -> (size(s)=w873:i32)
          n421 = Array Subset(array=w874, index=w873, length=w872) -> (w871:T7[])
          n422 = Build Array (concatenate)(w876, w878, w871) -> (w877:T7[])
        }
      }
      "Analysis Info cluster" <- w865
    }
  }
